vi "Template Change Template INI File.vi"(8 "error in (no error)":errorcluster, 11 "Template Record":T1) -> (0 "error out":errorcluster)   [LabVIEW 2011]
uses:
  Template Record.ctl
  <vilib>/Utility/config.llb/Read Key (String).vi
  <vilib>/Utility/config.llb/Write Key (String).vi
  <vilib>/Utility/config.llb/NI_LVConfig.lvlib
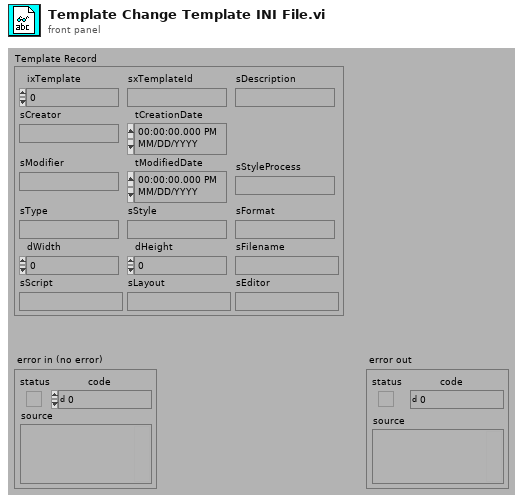
[diagram p1: front panel]
types:
  T1 = typedef "Template Record.ctl" = cluster{"ixTemplate":i32, "sxTemplateId":string, "sDescription":string, "sCreator":string, "tCreationDate":timestamp, "sModifier":string, "tModifiedDate":timestamp, "sType":string, "sStyle":string, "sFormat":string, "dWidth":dbl, "dHeight":dbl, "sFilename":string, "sScript":string, "sLayout":string, "sEditor":string, "sStyleProcess":string}
  T2 = typedef "NI_LVConfig.lvlib/Config Data RefNum.ctl" = refnum<k1>
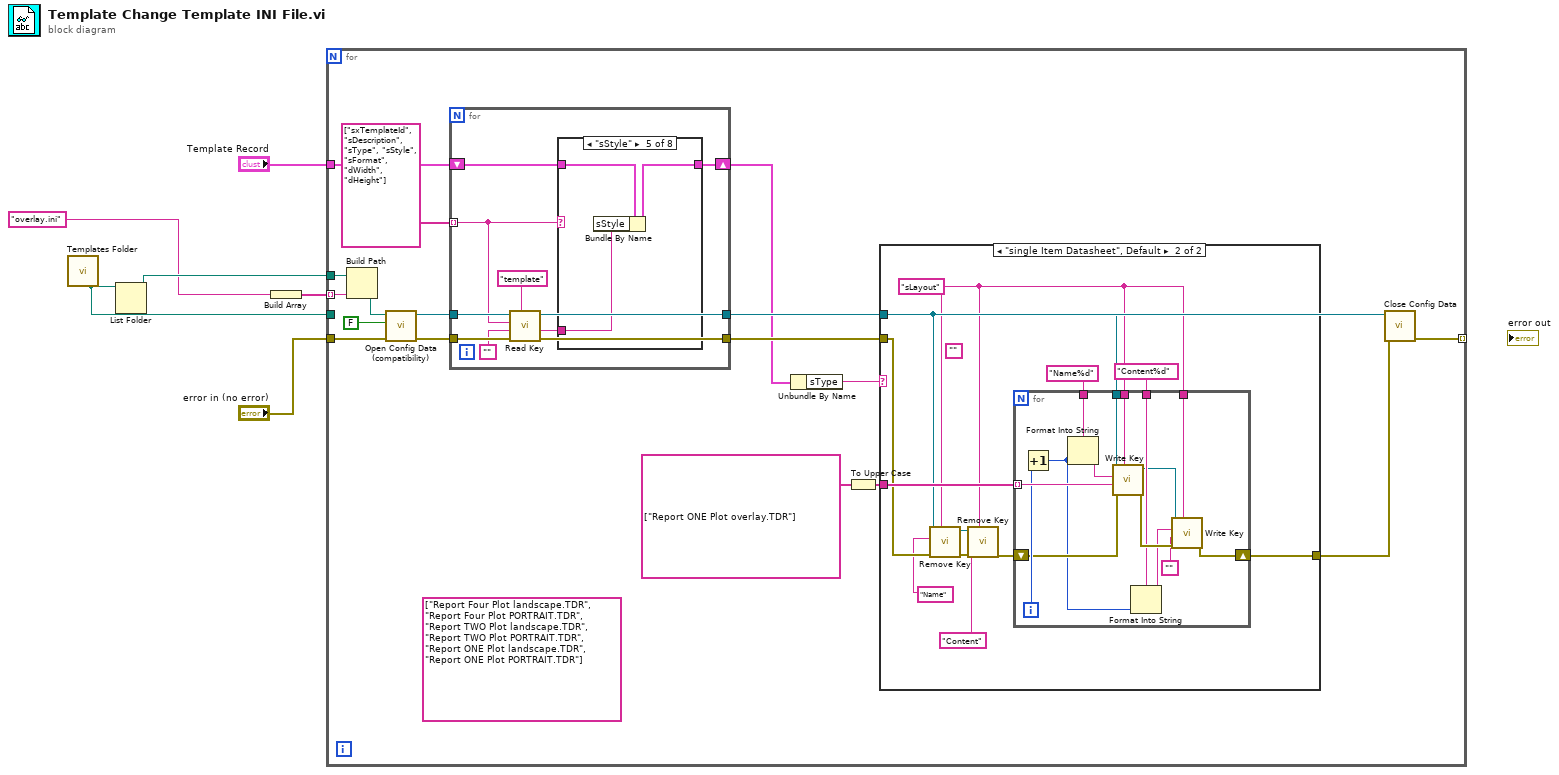
[diagram p0: block diagram]
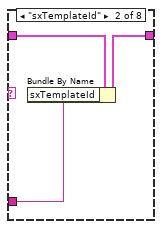
[diagram p4: hidden frame]
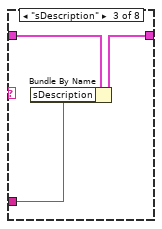
[diagram p5: hidden frame]
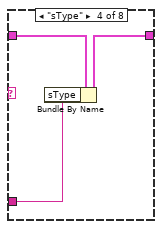
[diagram p6: hidden frame]
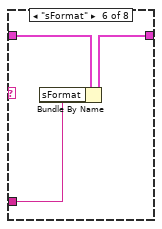
[diagram p7: hidden frame]
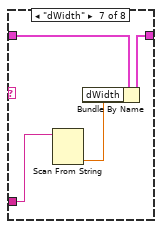
[diagram p8: hidden frame]
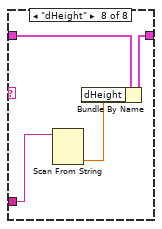
[diagram p9: hidden frame]
diagram:
  n1 = call "Templates Folder.vi"() -> ("Templates Folder"=w3:path)  [unwired: 1 in, 2 out]
  n2 = List Folder(path=w3) -> (path out=w4:path)  [unwired: 1 in, 5 out]
  n3 = Build Array("overlay.ini" ("pattern")) -> (w1:string[])
  n4 = for {
    tunnel: "Template Record" -> [w20]
    tunnel: "error in (no error)" -> [w18]
    tunnel: [w12] -> _ mode=indexing
    tunnel: w1 -> [w10] mode=indexing
    tunnel: w4 -> [w11]
    tunnel: w3 -> [_]
    (unwired) string[] ["Report Four Plot landscape.TDR", "Report Four Plot PORTRAIT.TDR", "Report TWO Plot landscape.TDR", "Report TWO Plot PORTRAIT.TDR", "Report ONE Plot landscape.TDR", "Report ONE Plot PORTRAIT.TDR"]
    n5 = Build Path(base path=w11, name or relative path=w10) -> (appended path=w7:path)
    n6 = call <vilib>:"Open Config Data (compatibility).vi"("error in (no error)"=w18, "create file if necessary (T)"=FALSE, "configuration file path"=w7) -> ("error out"=w22:errorcluster, "refnum"=w21:T2)  [unwired: 6 in, 1 out]
    n7 = for {
      tunnel: w22 -> [w61]
      tunnel: string[] ["sxTemplateId", "sDescription", "sType", "sStyle", "sFormat", "dWidth", "dHeight"] -> [w54] mode=indexing
      tunnel: [w59] -> w17
      tunnel: w21 -> [w58]
      shift-right: [w56] -> w14
      shift-left: w20 -> [w57]
      tunnel: [w53] -> w15
      n8 = call-poly <vilib>:"Read Key.vi"("section"="template", "error in (no error)"=w61, "default value"="", "key"=w54, "refnum"=w58) -> ("error out"=w59:errorcluster, "value"=w52:string, "refnum out"=w53:T2)  [unwired: 1 in, 3 out]
      n9 = case shown="\"sStyle\"" w54 {
        tunnel: w57 -> [w62 w65 w68 w71 w74 w77 w81 w85]
        tunnel: [w62 w64 w67 w70 w73 w76 w80 w84] -> w56
        tunnel: w52 -> [_ w63 w66 w69 w72 w75 w79 w83]
        frame "unknown", Default {
        }
        frame "sxTemplateId" {
          n10 = Bundle By Name(cluster=w65, "sxTemplateId"=w63) -> (w64:T1)
        }
        frame "sDescription" {
          n11 = Bundle By Name(cluster=w68, "sDescription"=w66) -> (w67:T1)
        }
        frame "sType" {
          n12 = Bundle By Name(cluster=w71, "sType"=w69) -> (w70:T1)
        }
        frame "sStyle" {
          n13 = Bundle By Name(cluster=w74, "sStyle"=w72) -> (w73:T1)
        }
        frame "sFormat" {
          n14 = Bundle By Name(cluster=w77, "sFormat"=w75) -> (w76:T1)
        }
        frame "dWidth" {
          n15 = Scan From String(input string=w79) -> (output 1=w78:dbl)  [unwired: 3 in, 4 out]
          n16 = Bundle By Name(cluster=w81, "dWidth"=w78) -> (w80:T1)
        }
        frame "dHeight" {
          n17 = Scan From String(input string=w83) -> (output 1=w82:dbl)  [unwired: 3 in, 4 out]
          n18 = Bundle By Name(cluster=w85, "dHeight"=w82) -> (w84:T1)
        }
      }
    }
    n19 = Unbundle By Name(w14) -> ("sType"=w13:string)
    n20 = To Upper Case(1:string[] ["Report ONE Plot overlay.TDR"]) -> (0:w9:string[])
    n21 = case shown="\"single Item Datasheet\", Default" w13 {
      tunnel: w9 -> [_ w36]
      tunnel: w17 -> [w24 w27]
      tunnel: [w24 w34] -> w16
      tunnel: w15 -> [_ w28]
      frame "False" {
      }
      frame "single Item Datasheet", Default {
        (unwired) ""
        w32 = "sLayout" ("section")
        n22 = call <vilib>:"Remove Key.vi"("section"=w32, "error in (no error)"=w27, "key"="Name" ("section"), "refnum"=w28) -> ("error out"=w30:errorcluster, "refnum out"=w29:T2)  [unwired: 6 out]
        n23 = call <vilib>:"Remove Key.vi"("section"=w32, "error in (no error)"=w30, "key"="Content" ("section"), "refnum"=w29) -> ("error out"=w31:errorcluster)  [unwired: 7 out]
        n24 = for {
          tunnel: w28 -> [w51]
          tunnel: w32 -> [w50]
          tunnel: w36 -> [w49] mode=indexing
          tunnel: "Name%d" ("section") -> [w48]
          shift-right: [w44] -> w34
          shift-left: w31 -> [w45]
          tunnel: "Content%d" ("section") -> [w42]
          tunnel: w32 -> [w40]
          i -> [w46]
          n25 = Increment(x=w46) -> (x+1=w41:i32)
          n26 = Format Into String(format string=w48, w41) -> (resulting string=w47:string)  [unwired: 2 in, 1 out]
          n27 = call-poly <vilib>:"Write Key.vi"("section"=w50, "error in (no error)"=w45, "value"=w49, "key"=w47, "refnum"=w51) -> ("error out"=w43:errorcluster, "refnum out"=w39:T2)  [unwired: 1 in, 4 out]
          n28 = Format Into String(format string=w42, w41) -> (resulting string=w38:string)  [unwired: 2 in, 1 out]
          n29 = call-poly <vilib>:"Write Key.vi"("section"=w40, "error in (no error)"=w43, "value"="", "key"=w38, "refnum"=w39) -> ("error out"=w44:errorcluster)  [unwired: 1 in, 5 out]
        }
      }
    }
    n30 = call <vilib>:"Close Config Data.vi"("error in (no error)"=w16, "refnum"=w15) -> ("error out"=w12:errorcluster)  [unwired: 1 in, 8 out]
  }
